vi "Init Camera.vi"(7 "error in 2":errorcluster caption="error in") -> (0 "error out":errorcluster, 1 "session out":T1)   [LabVIEW 2017]
uses:
  <vilib>/userdefined/High Color/IMAQdx.ctl
  <vilib>/vision/driver/NI_Vision_Acquisition_Software.lvlib
  <resource>/objmgr/imaqdx.rc
panel:
  in  "Exposure::Mode 3":u32(ring) caption="Brightness::Mode" items=["Manual"]
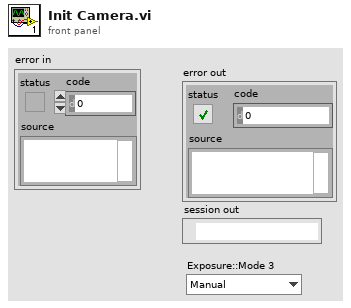
[diagram p1: front panel]
types:
  T1 = typedef "IMAQdx.ctl" = refnum<k21>
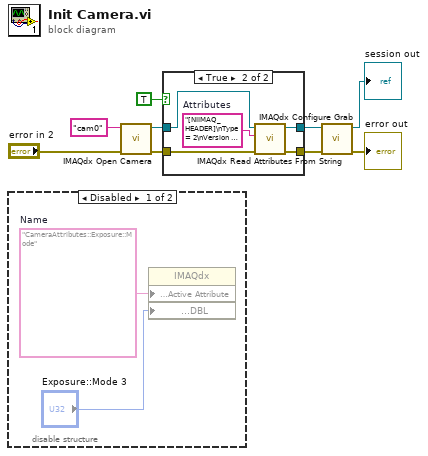
[diagram p0: block diagram]
diagram:
  n1 = disable-structure shown="Disabled" {
    frame Disabled {
      w14 = "CameraAttributes::Exposure::Mode"  # Name
      n2 = property class="IMAQdx"("Camera Attributes:Active Attribute"=w14, "Camera Attributes:Value:DBL"="Exposure::Mode 3") -> (reference=w13:T1, error in=w12:errorcluster, error out=w11:errorcluster)  [unwired: 1 out]
    }
    frame Enabled {
    }
  }
  n3 = call <vilib>:"IMAQdx Open Camera.vi"("error in"="error in 2", "Session In"="cam0" ("Interface Name")) -> ("error out"=w4:errorcluster, "Session Out"=w5:T1)  [unwired: 1 in, 7 out]
  n4 = case shown="True" TRUE ("Init Attributes") {
    tunnel: w5 -> [w16 w21]
    tunnel: w4 -> [w15 w19]
    tunnel: [w16 w18] -> w2
    tunnel: [w15 w17] -> w1
    frame False {
    }
    frame True {
      w20 = "[NIIMAQ_HEADER]\nType = 2\nVersion = 8\n\n[CAMERA_DATA]\nAcquisitionAttributes::Bayer::Algorithm = \"Bilinear\"\nAcquisitionAttributes::Bayer::GainB = \"1\"\nAcquisitionAttributes::Bayer::GainG = \"1\"\nAcquisitionAttributes::Bayer::GainR = \"1\"\nAcquisitionAttributes::Bayer::Pattern = \"Use hardware value\"\nAcquisitionAttributes::BitsPerPixel = \"Use hardware value\"\nAcquisitionAttributes::IgnoreFirstFrame = \"false\"\nAcquisitionAttributes::ImageDecoderCopyMode = \"Auto\"\nAcquisitionAttributes::OutputImageType = \"Auto\"\nAcquisitionAttributes::OverwriteMode = \"Get Newest\"\nAcquisitionAttributes::PixelSignedness = \"Use hardware value\"\nAcquisitionAttributes::ReceiveTimestampMode = \"None\"\nAcquisitionAttributes::ShiftPixelBits = \"false\"\nAcquisitionAttributes::SwapPixelBytes = \"false\"\nAcquisitionAttributes::Timeout = \"5000\"\nAcquisitionAttributes::VideoMode = \"160 x 120 YUY 2 30.00 fps\"\nCameraAttributes::BacklightCompensation::Mode = \"Manual\"\nCameraAttributes::BacklightCompensation::Value = \"1\"\nCameraAttributes::Brightness::Mode = \"Manual\"\nCameraAttributes::Brightness::Value = \"128\"\nCameraAttributes::Contrast::Mode = \"Manual\"\nCameraAttributes::Contrast::Value = \"32\"\nCameraAttributes::Exposure::Mode = \"Manual\"\nCameraAttributes::Exposure::Value = \"249\"\nCameraAttributes::Focus::Mode = \"Auto\"\nCameraAttributes::Gain::Mode = \"Manual\"\nCameraAttributes::Gain::Value = \"64\"\nCameraAttributes::Pan::Mode = \"Manual\"\nCameraAttributes::Pan::Value = \"0\"\nCameraAttributes::PowerLineFrequency::Mode = \"60Hz\"\nCameraAttributes::Saturation::Mode = \"Manual\"\nCameraAttributes::Saturation::Value = \"32\"\nCameraAttributes::Sharpness::Mode = \"Manual\"\nCameraAttributes::Sharpness::Value = \"22\"\nCameraAttributes::Tilt::Mode = \"Manual\"\nCameraAttributes::Tilt::Value = \"0\"\nCameraAttributes::WhiteBalance::Mode = \"Manual\"\nCameraAttributes::WhiteBalance::Value = \"4877\"\nCameraAttributes::Zoom::Mode = \"Manual\"\nCameraAttributes::Zoom::Value = \"1\"\n"  # Attributes
      n5 = call <vilib>:"IMAQdx Read Attributes From String.vi"("error in"=w19, "Attributes String In"=w20, "Session In"=w21) -> ("error out"=w17:errorcluster, "Session Out"=w18:T1)  [unwired: 7 out]
    }
  }
  n6 = call <vilib>:"IMAQdx Configure Grab.vi"("error in"=w1, "Session In"=w2) -> ("error out"=→"error out":errorcluster, "Session Out"=→"session out":T1)  [unwired: 8 out]
